vi "IAmGLF-DeleteDVR.vi"(8 "error in (no error)":errorcluster, 11 "View in":refnum<class "View.lvclass">) -> (0 "error out":errorcluster, 3 "View out":refnum<class "View.lvclass">)   [LabVIEW 2024, in "GLF.lvlib" / "View.lvclass"]
doc: "<B>Summary</B>\nTo delete the class DVR from standalone process."
uses:
  View.lvclass
  View.lvclass/View.ctl
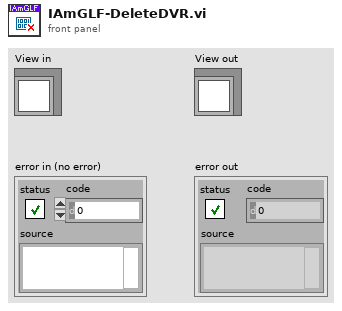
[diagram p1: front panel]
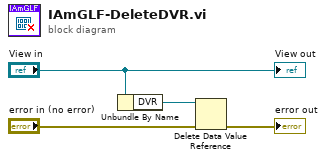
[diagram p0: block diagram]
diagram:
  n1 = Unbundle By Name("View in") -> ("DVR"=w3:refnum<data-value>)
  n2 = Delete Data Value Reference(data value reference=w3, error in="error in (no error)") -> (error out=→"error out":errorcluster)  [unwired: 1 out]
  "View out" <- "View in"
